vi "Plot Names Tester.vi"() -> ()   [LabVIEW 2010]
doc: "This VI is used to test the Set Plot Names VI."
panel:
  in  "Plot Names":string[](array[string])
  out "Waveform Graph":dbl[](graph)
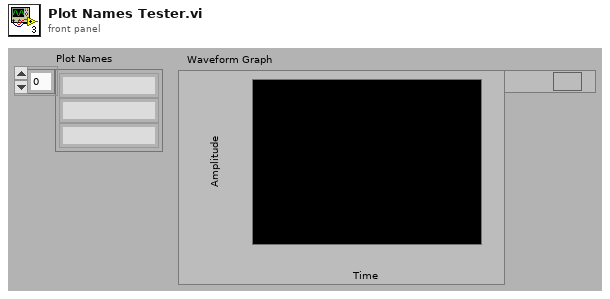
[diagram p1: front panel]
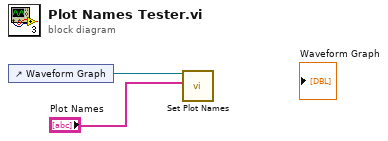
[diagram p0: block diagram]
diagram:
  n1 = control-ref of="Waveform Graph"() -> (w1:refnum<vi>)
  n2 = call "Set Plot Names.vi"("Plot Names"="Plot Names", "Graph Reference"=w1) -> ()  [unwired: 9 in, 1 out]
